vi "Result.Measurements Status Check.vi"(11 "Meas":T1[](array[typedef]) {"Status" items=["LOG", "PASS", "FAIL", "ERROR"]}) -> (2 "Failing":bool, 3 "Failing Items":T1[](array[typedef]) {"Status" items=["LOG", "PASS", "FAIL", "ERROR"]})   [LabVIEW 2019]
uses:
  Result.Measurement Item.ctl
  Result.Measurement and Attribute Item Status.ctl
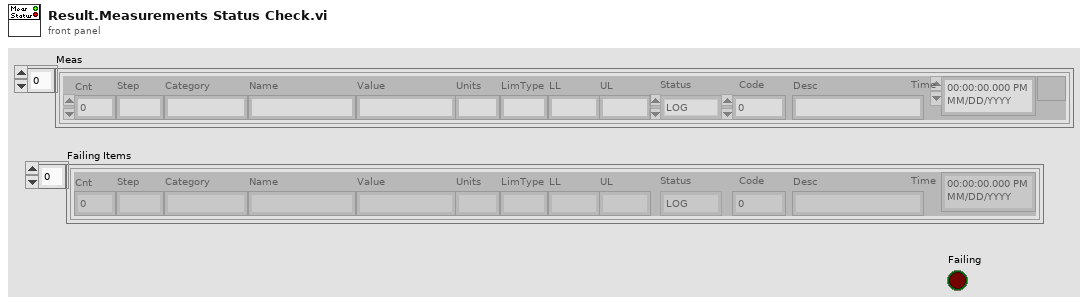
[diagram p1: front panel]
types:
  T1 = typedef "Result.Measurement Item.ctl" = cluster{"Cnt":i32, "Step":string, "Category":string, "Name":string, "Value":string, "Units":string, "LimType":string, "LL":string, "UL":string, "Status":T2, "Code":i32, "Desc":string, "Time":timestamp}
  T2 = typedef "Result.Measurement and Attribute Item Status.ctl" = i32
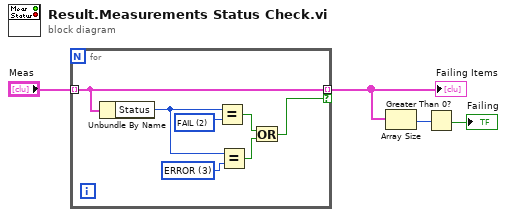
[diagram p0: block diagram]
diagram:
  n1 = for {
    tunnel: "Meas" -> [w11] mode=indexing
    tunnel: [w11] -> w3 mode=indexing if=w5
    w8 = T2 3 items=["LOG", "PASS", "FAIL", "ERROR"] ("y")
    w9 = T2 2 items=["LOG", "PASS", "FAIL", "ERROR"] ("y")
    n2 = Unbundle By Name(w11) -> ("Status"=w10:T2)
    n3 = Equal?(x=w10, y=w9) -> (x = y?=w7:bool)
    n4 = Equal?(x=w10, y=w8) -> (x = y?=w6:bool)
    n5 = Or(x=w7, y=w6) -> (x .or. y?=w5:bool)
  }
  "Failing Items" <- w3
  n6 = Array Size(array=w3) -> (size(s)=w2:i32)
  n7 = Greater Than 0?(x=w2) -> (x > 0?=→"Failing":bool)
